vi "raddrizzatore_unipolare.vi"(2 "waveform":waveform(dbl)) -> (0 "output waveform":waveform(dbl))   [LabVIEW 2009]
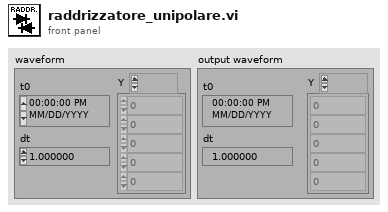
[diagram p1: front panel]
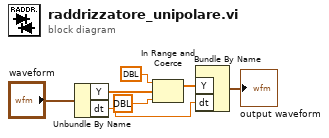
[diagram p0: block diagram]
diagram:
  n1 = Unbundle By Name("waveform") -> ("Y"=w6:dbl[], "dt"=w4:dbl)
  n2 = In Range and Coerce(upper limit=dbl ?, x=w6, lower limit=dbl ?) -> (coerced(x)=w5:dbl[])  [unwired: 1 out]
  n3 = Bundle By Name("Y"=w5, "dt"=w4) -> (→"output waveform":waveform(dbl))  [unwired: 1 in]
